vi "Actor Core.vi"(8 "error in":errorcluster, 11 "[V] Login in":refnum<class "[V] Login.lvclass">) -> (0 "error out":errorcluster, 3 "Actor out":refnum<class "Actor.lvclass">)   [LabVIEW 2020, in "[V] Login.lvlib" / "[V] Login.lvclass"]
doc: "(<B>Filename</B>: Actor Framework.lvlib:Actor.lvclass:Actor Core.vi)\n\nReceives messages to the actor, reacts to them, and initiates any error handling that may shut the actor down.\n\nDescendant classes may override this VI to append parallel tasks for the actor to complete while it handles messages. Overrides use the Call Parent Class Method node."
uses:
  [V] Login.lvclass
  <vilib>/ActorFramework/Actor/Actor.lvclass
  C:/Program Files/National Instruments/LabVIEW 2020/vi.lib/ActorFramework/Actor/Actor.lvclass
  Control/rmb checkbox.ctl
  Control/login.ctl
  Control/ring arrow.ctl
  <vilib>/ActorFramework/Actor/Actor.lvclass/Actor.ctl
  <vilib>/ActorFramework/Message Enqueuer/Message Enqueuer.lvclass/Message Enqueuer.ctl
  [V] Login.lvclass/[V] Login.ctl
  [V] Login Messages/Event Select User Msg/Event Select User Msg.lvclass/Event Select User Msg.ctl
  INF of [V] Login Messages/Login Rmb User Msg/Login Rmb User Msg.lvclass/Login Rmb User Msg.ctl
  <vilib>/ActorFramework/Message Enqueuer/Init from Existing Queue.vi
  <vilib>/ActorFramework/Message Enqueuer/Enqueue.vi
  <vilib>/ActorFramework/Stop Msg/Stop Msg.lvclass
  C:/Program Files/National Instruments/LabVIEW 2020/vi.lib/ActorFramework/Message/Message.lvclass
  [V] Login Messages/Event Expand User Msg/Event Expand User Msg.lvclass
  [V] Login Messages/Event Contract User Msg/Event Contract User Msg.lvclass
  [V] Login Messages/Event Select User Msg/Event Select User Msg.lvclass
  INF of [V] Login Messages/Login Rmb User Msg/Login Rmb User Msg.lvclass
  [V] Login Messages/Event Login Msg/Event Login Msg.lvclass
  <vilib>/ActorFramework/Message Priority Queue/Priority Enqueue.vi
  <vilib>/ActorFramework/Message Enqueuer/Message Enqueuer.lvclass
panel:
  in  "user ring arrow":T1
  out "error msg":string
  in  "login":T2
  in  "rmb user":T3 caption="记住用户名"
  in  "pwd":string
  out "pwd tip":string="请输入密码"
  in  "user":string
  out "user tip":string="请输入用户名"
  out "title":string
  in  "user list":i32(listbox)
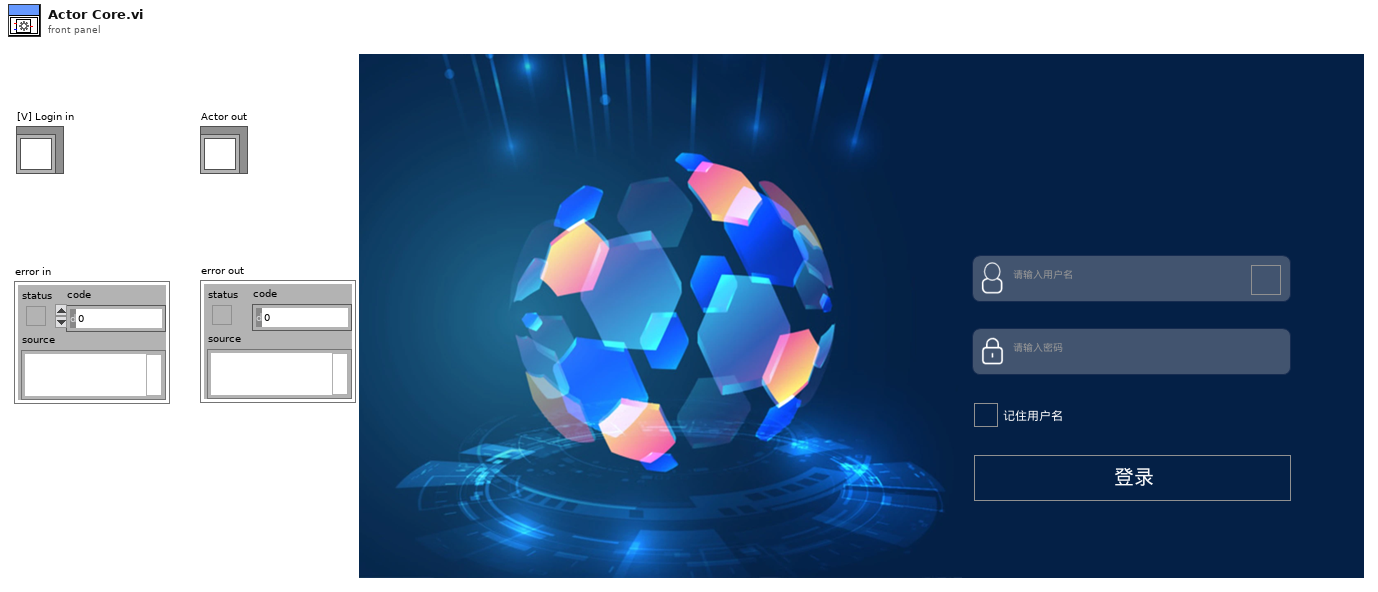
[diagram p1: front panel]
types:
  T1 = typedef "[V] Login.lvlib/[V] Login.lvclass/ring arrow.ctl" = bool
  T2 = typedef "[V] Login.lvlib/[V] Login.lvclass/login.ctl" = bool
  T3 = typedef "[V] Login.lvlib/[V] Login.lvclass/rmb checkbox.ctl" = bool
  T4 = typedef "LVPoint32TypeDef.ctl" = cluster{"Horizontal":i32, "Vertical":i32}
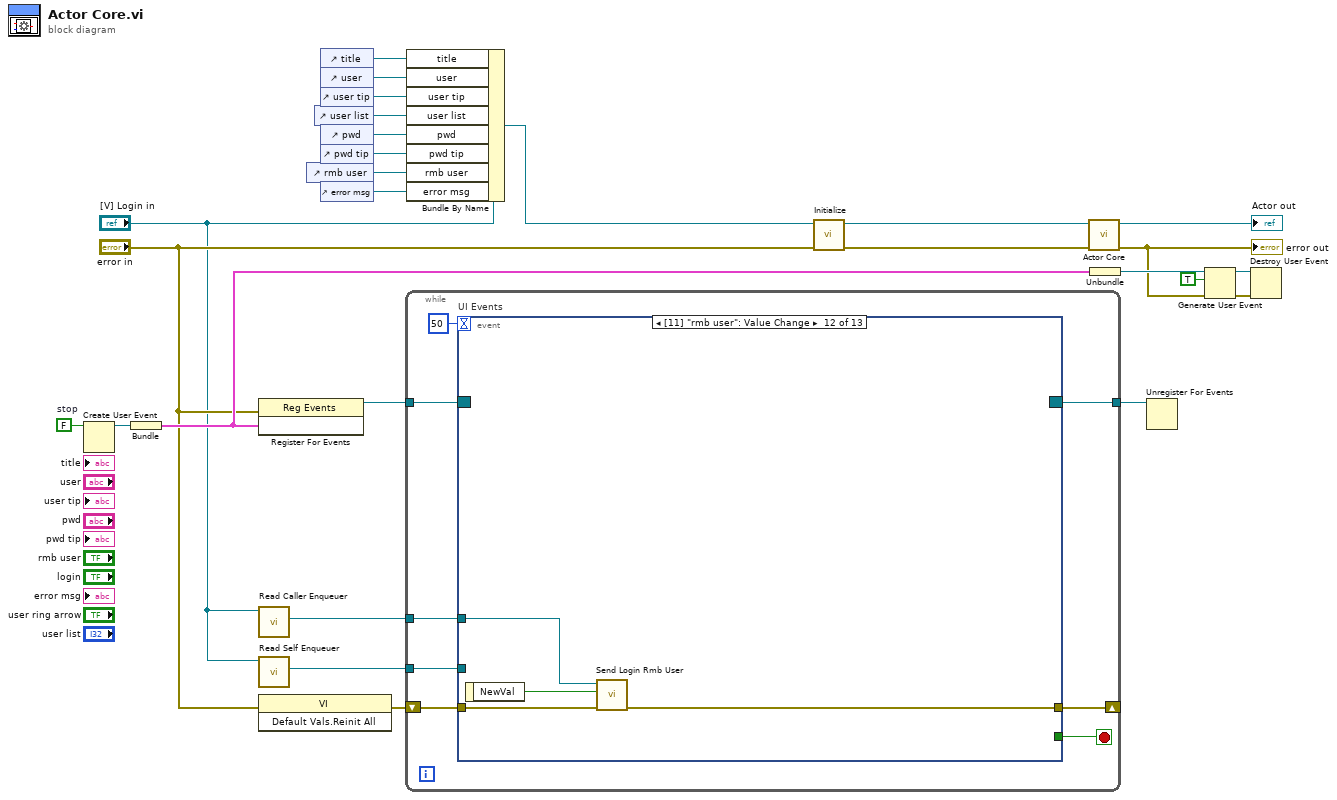
[diagram p0: block diagram]
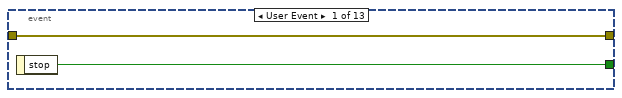
[diagram p2: hidden frame]
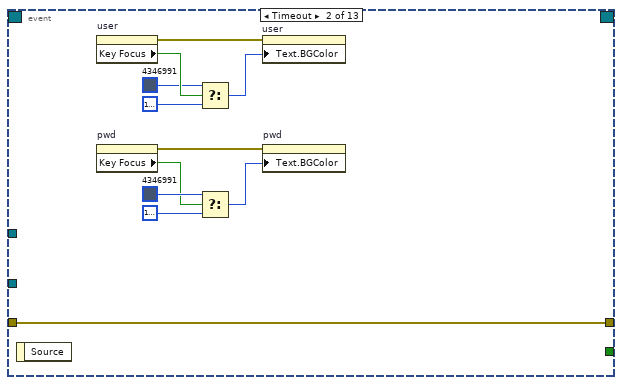
[diagram p3: hidden frame]
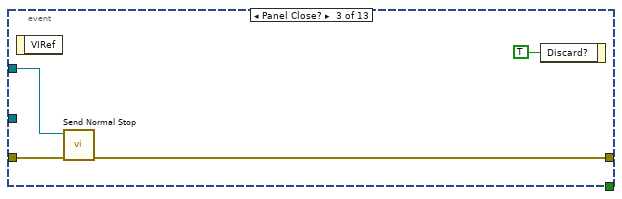
[diagram p4: hidden frame]
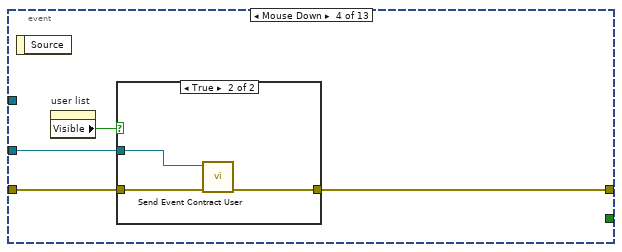
[diagram p5: hidden frame]
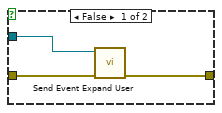
[diagram p6: hidden frame]
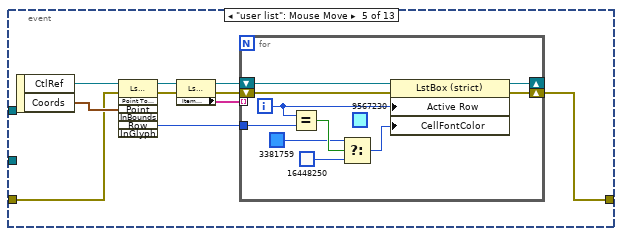
[diagram p7: hidden frame]
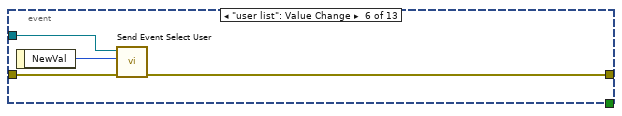
[diagram p8: hidden frame]
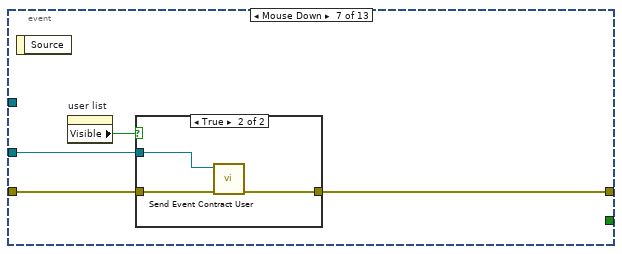
[diagram p9: hidden frame]
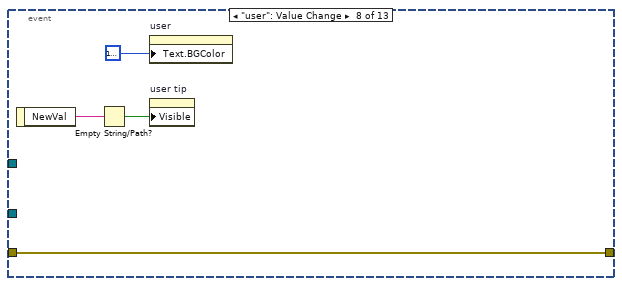
[diagram p11: hidden frame]
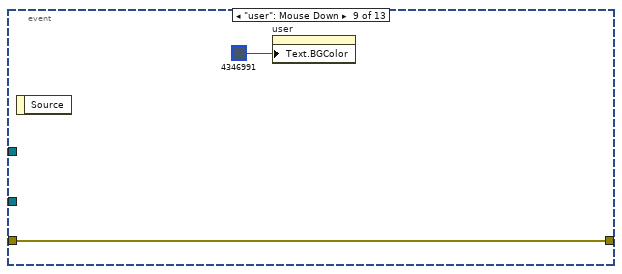
[diagram p12: hidden frame]
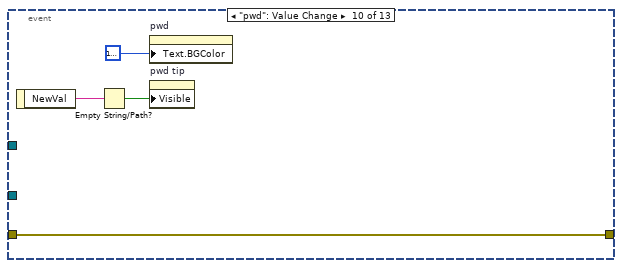
[diagram p13: hidden frame]
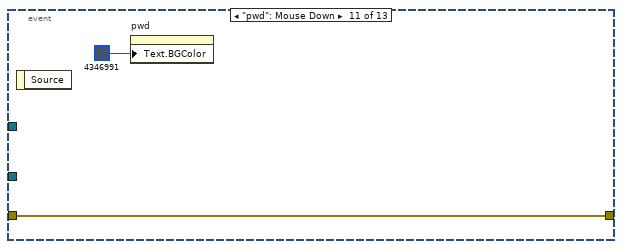
[diagram p14: hidden frame]
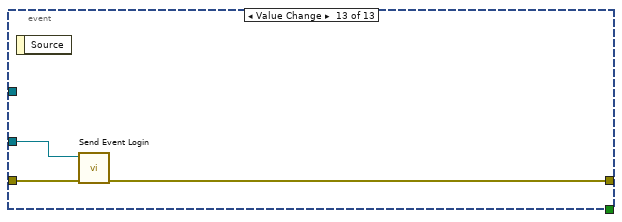
[diagram p15: hidden frame]
diagram:
  w20 = FALSE  # stop
  n1 = Create User Event(user event datatype=w20) -> (user event=w23:refnum<user-event>)  [unwired: 1 in, 1 out]
  n2 = Bundle("stop"=w23) -> (w24:cluster{"stop":refnum<user-event>})  [unwired: 1 in]
  n3 = register-events ("Main Register for Events")(error in="error in", w24) -> (reference out=w15:refnum<event-registration>)  [unwired: 1 in, 1 out]
  n4 = call <vilib>:"Read Caller Enqueuer.vi"("Actor"="[V] Login in") -> ("Caller Enqueuer"=w18:refnum<class "Message Enqueuer.lvclass">)  [unwired: 10 in]
  n5 = call <vilib>:"Read Self Enqueuer.vi"("Actor"="[V] Login in") -> ("Self Enqueuer"=w17:refnum<class "Message Enqueuer.lvclass">)  [unwired: 10 in]
  n6 = invoke class="VI" method="Default Vals.Reinit All"(error in="error in") -> (error out=w19:errorcluster)  [unwired: 2 in, 2 out]
  n7 = control-ref of="rmb user"() -> (w2:refnum<vi>)
  n8 = control-ref of="user list"() -> (w5:refnum<vi>)
  n9 = control-ref of="title"() -> (w8:refnum<vi>)
  n10 = control-ref of="user"() -> (w7:refnum<vi>)
  n11 = control-ref of="user tip"() -> (w6:refnum<vi>)
  n12 = control-ref of="pwd"() -> (w4:refnum<vi>)
  n13 = control-ref of="pwd tip"() -> (w3:refnum<vi>)
  n14 = control-ref of="error msg"() -> (w1:refnum<vi>)
  n15 = while {
    tunnel: w15 -> [w35]
    tunnel: [w33] -> w16
    tunnel: w17 -> [w32]
    tunnel: w18 -> [w29]
    shift-right: [w30] -> _
    shift-left: w19 -> [w31]
    stop <- w34 stop-if-true
    n16 = event "UI Events" shown="[11] \"rmb user\": Value Change" {
      selector: w35 -> [_ _ _ _ _ _ _ _ _ _ _ _ _]
      dyn-events: [_ _ _ _ _ _ _ _ _ _ _ _ _] -> w33
      timeout: 50 -> [_ _ _ _ _ _ _ _ _ _ _ _ _]
      tunnel: [w36 _ _ _ _ _ _ _ _ _ _ _ _] -> w34
      tunnel: w32 -> [_ _ _ w54 _ w85 w89 _ _ _ _ _ w112]
      tunnel: w31 -> [w37 w38 w51 w56 w70 w86 w90 w96 w100 w102 w106 w110 w113]
      tunnel: [w37 w38 w50 w53 w63 w84 w87 w96 w100 w102 w106 w107 w111] -> w30
      tunnel: w29 -> [_ _ w49 _ _ _ _ _ _ _ _ w109 _]
      event User Event {
        n17 = event-data() -> ("stop"=w36:bool)  [unwired: 1 in]
      }
      event Timeout {
        n18 = event-data() -> ()  [unwired: 1 in, 1 out]
        n19 = property on="user" class="Str"() -> (error out=w48:errorcluster, "Key Focus"=w47:bool)  [unwired: 2 in, 1 out]
        n20 = property on="pwd" class="Str"() -> (error out=w39:errorcluster, "Key Focus"=w40:bool)  [unwired: 2 in, 1 out]
        n21 = Select(t=u32 4346991 ("Text.Text Colors:Text Color"), s=w47, f=u32 16777216 ("Text.Text Colors:Text Color")) -> (s? t:f=w44:u32)
        n22 = Select(t=u32 4346991 ("Text.Text Colors:Text Color"), s=w40, f=u32 16777216 ("Text.Text Colors:Text Color")) -> (s? t:f=w43:u32)
        n23 = property on="user" class="Str"(error in=w48, "Text.BGColor"=w44) -> ()  [unwired: 1 in, 2 out]
        n24 = property on="pwd" class="Str"(error in=w39, "Text.BGColor"=w43) -> ()  [unwired: 1 in, 2 out]
      }
      event Panel Close? {
        n25 = event-data() -> ()  [unwired: 1 in, 1 out]
        n26 = call <vilib>:"Send Normal Stop.vi"("error in (no error)"=w51, "Message Enqueuer"=w49) -> ("error out"=w50:errorcluster)  [unwired: 9 in]
        n27 = event-data("Discard?"=TRUE) -> ()  [unwired: 1 in, 1 out]
      }
      event Mouse Down {
        n28 = event-data() -> ()  [unwired: 1 in, 1 out]
        n29 = property on="user list" class="LstBox (strict)"() -> ("Visible"=w55:bool)  [unwired: 2 in, 2 out]
        n30 = case shown="True" w55 {
          tunnel: w56 -> [w59 w62]
          tunnel: w54 -> [w58 w60]
          tunnel: [w57 w61] -> w53
          frame False {
            n31 = call "Send Event Expand User.vi"("error in (no error)"=w59, "Message Enqueuer"=w58) -> ("error out"=w57:errorcluster)  [unwired: 8 in, 1 out]
          }
          frame True {
            n32 = call "Send Event Contract User.vi"("error in (no error)"=w62, "Message Enqueuer"=w60) -> ("error out"=w61:errorcluster)  [unwired: 8 in, 1 out]
          }
        }
      }
      event "user list": Mouse Move {
        n33 = event-data() -> ("CtlRef"=w72:refnum<vi>, "Coords"=w71:T4)  [unwired: 1 in]
        n34 = invoke class="LstBox (strict)" method="Point To Row"(reference=w72, error in=w70, "Point"=w71) -> (reference out=w68:refnum<vi>, error out=w69:errorcluster, "Row"=w67:i32)  [unwired: 4 in, 4 out]
        n35 = property class="LstBox (strict)"(reference=w68, error in=w69) -> (reference out=w64:refnum<vi>, error out=w65:errorcluster, "Item Names"=w66:string[])
        n36 = for {
          tunnel: w67 -> [w78]
          tunnel: w66 -> [_] mode=indexing
          shift-right: [w79] -> w63
          shift-left: w65 -> [w82]
          shift-right: [w80] -> _
          shift-left: w64 -> [w81]
          i -> [w77]
          (unwired) u32 9567230 ("活动行:单元格字体:颜色")
          n37 = Equal?(x=w77, y=w78) -> (x = y?=w75:bool)
          n38 = Select(t=u32 3381759 ("活动行:单元格字体:颜色"), s=w75, f=u32 16448250 ("活动行:单元格字体:颜色")) -> (s? t:f=w76:u32)
          n39 = property class="LstBox (strict)"(reference=w81, error in=w82, "Active Row"=w77, "CellFontColor"=w76) -> (reference out=w80:refnum<vi>, error out=w79:errorcluster)
        }
      }
      event "user list": Value Change {
        n40 = event-data() -> ("NewVal"=w83:i32)  [unwired: 1 in]
        n41 = call "Send Event Select User.vi"("error in (no error)"=w86, "index"=w83, "Message Enqueuer"=w85) -> ("error out"=w84:errorcluster)  [unwired: 7 in, 1 out]
      }
      event Mouse Down {
        n42 = event-data() -> ()  [unwired: 1 in, 1 out]
        n43 = property on="user list" class="LstBox (strict)"() -> ("Visible"=w88:bool)  [unwired: 2 in, 2 out]
        n44 = case shown="True" w88 {
          tunnel: w90 -> [w91 w94]
          tunnel: w89 -> [_ w93]
          tunnel: [w91 w92] -> w87
          frame False {
          }
          frame True {
            n45 = call "Send Event Contract User.vi"("error in (no error)"=w94, "Message Enqueuer"=w93) -> ("error out"=w92:errorcluster)  [unwired: 8 in, 1 out]
          }
        }
      }
      event "user": Value Change {
        n46 = event-data() -> ("NewVal"=w98:string)  [unwired: 1 in]
        n47 = Empty String/Path?(string/path=w98) -> (empty?=w97:bool)
        n48 = property on="user" class="Str"("Text.BGColor"=u32 16777216 ("Text.Text Colors:Text Color")) -> ()  [unwired: 2 in, 2 out]
        n49 = property on="user tip" class="Str"("Visible"=w97) -> ()  [unwired: 2 in, 2 out]
      }
      event "user": Mouse Down {
        n50 = event-data() -> ()  [unwired: 1 in, 1 out]
        n51 = property on="user" class="Str"("Text.BGColor"=u32 4346991 ("Text.Text Colors:Text Color")) -> ()  [unwired: 2 in, 2 out]
      }
      event "pwd": Value Change {
        n52 = event-data() -> ("NewVal"=w104:string)  [unwired: 1 in]
        n53 = Empty String/Path?(string/path=w104) -> (empty?=w103:bool)
        n54 = property on="pwd" class="Str"("Text.BGColor"=u32 16777216 ("Text.Text Colors:Text Color")) -> ()  [unwired: 2 in, 2 out]
        n55 = property on="pwd tip" class="Str"("Visible"=w103) -> ()  [unwired: 2 in, 2 out]
      }
      event "pwd": Mouse Down {
        n56 = event-data() -> ()  [unwired: 1 in, 1 out]
        n57 = property on="pwd" class="Str"("Text.BGColor"=u32 4346991 ("Text.Text Colors:Text Color")) -> ()  [unwired: 2 in, 2 out]
      }
      event Value Change {
        n58 = event-data() -> ("NewVal"=w108:T3)  [unwired: 1 in]
        n59 = call "Send Login Rmb User.vi"("error in (no error)"=w110, "rmb user"=w108, "Message Enqueuer"=w109) -> ("error out"=w107:errorcluster)  [unwired: 7 in, 1 out]
      }
      event Value Change {
        n60 = event-data() -> ()  [unwired: 1 in, 1 out]
        n61 = call "Send Event Login.vi"("error in (no error)"=w113, "Message Enqueuer"=w112) -> ("error out"=w111:errorcluster)  [unwired: 8 in, 1 out]
      }
    }
  }
  n62 = Bundle By Name(cluster="[V] Login in", "title"=w8, "user"=w7, "user tip"=w6, "user list"=w5, "pwd"=w4, "pwd tip"=w3, "rmb user"=w2, "error msg"=w1) -> (w9:refnum<class "[V] Login.lvclass">)
  n63 = call "Initialize.vi"("error in (no error)"="error in", "[V] Login in"=w9) -> ("error out"=w13:errorcluster, "[V] Login out"=w12:refnum<class "[V] Login.lvclass">)  [unwired: 8 in]
  n64 = call-parent "Actor Core.vi"("error in"=w13, "Actor in"=w12) -> ("error out"=w14:errorcluster, "Actor out"=→"Actor out":refnum<class "Actor.lvclass">)  [unwired: 8 in]
  "error out" <- w14
  n65 = Unbundle(w24) -> ("stop"=w25:refnum<user-event>)
  n66 = Unregister For Events(event registration refnum=w16) -> ()  [unwired: 1 in, 1 out]
  n67 = Generate User Event(user event=w25, event data cluster=TRUE ("event data"), error in=w14) -> (user event out=w22:refnum<user-event>, error out=w26:errorcluster)  [unwired: 1 in]
  n68 = Destroy User Event(user event=w22, error in=w26) -> ()  [unwired: 1 out]
